vi "execute.vi"(8 "error in (no error)":errorcluster, 10 "ComponentData.lvclass":refnum<class "ComponentData.lvclass">, 11 "OffState in":refnum<class "StandbyState.lvclass">) -> (0 "error out":errorcluster, 2 "ComponentData.lvclass 2":refnum<class "ComponentData.lvclass">, 3 "OffState out":refnum<class "StandbyState.lvclass">)   [LabVIEW 2013, in "ComponentData.lvlib" / "StandbyState.lvclass"]
uses:
  <userlib>/Common/Component/common_application/RT/ComponentData/ComponentState/StandbyState/StandbyState.lvclass
  <userlib>/Common/Component/common_application/RT/ComponentData/ComponentData/ComponentData.lvclass
  <userlib>/Common/Component/common_application/RT/ComponentData/ComponentState/ComponentState/ComponentState.lvclass
  <userlib>/Common/Component/common_application/RT/ComponentData/componentStateValues.ctl
  <userlib>/Common/Component/common_application/RT/ComponentData/ComponentState/DisabledState/DisabledState.lvclass
  <userlib>/Common/Component/common_application/RT/ComponentData/ComponentState/OffState/OffState.lvclass
  <userlib>/Common/Component/common_application/RT/ComponentData/ApplicationHandler/ApplicationHandler.lvclass
  <userlib>/Common/Component/common_application/RT/ComponentData.lvlib
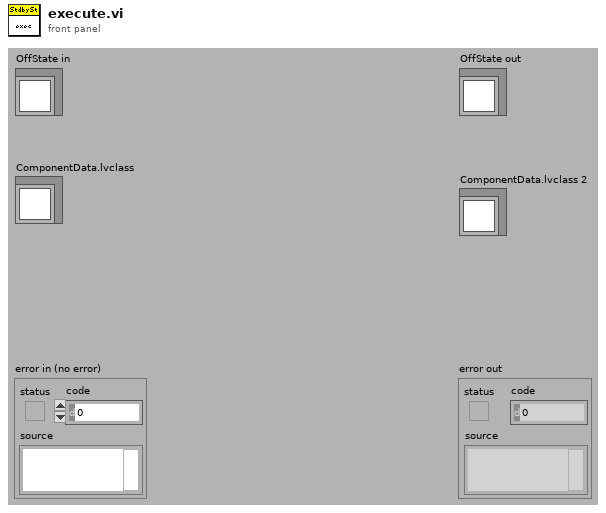
[diagram p1: front panel]
types:
  T1 = typedef "ComponentData.lvlib/componentStateValues.ctl" = enum16{"Off", "Standby", "Enabled", "Disabled", "Fault"}
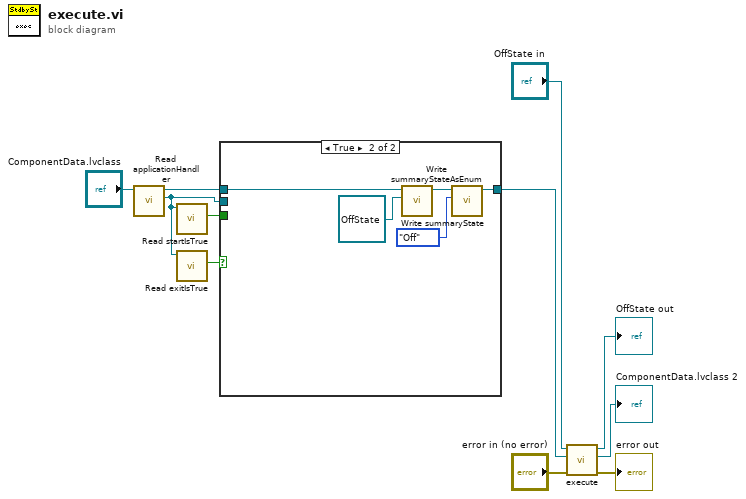
[diagram p0: block diagram]
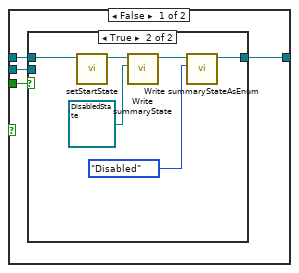
[diagram p2: hidden frame]
diagram:
  n1 = call <userlib>:"Read applicationHandler.vi"("ComponentData in"="ComponentData.lvclass") -> ("ApplicationHandler.lvclass"=w2:refnum<class "ApplicationHandler.lvclass">, "ComponentData out"=w4:refnum<class "ComponentData.lvclass">)  [unwired: 9 in]
  n2 = call <userlib>:"Read startIsTrue.vi"("ApplicationHandler in"=w2) -> ("startIsTrue"=w5:bool)  [unwired: 9 in, 1 out]
  n3 = call <userlib>:"Read exitIsTrue.vi"("ApplicationHandler in"=w2) -> ("exitIsTrue"=w1:bool)  [unwired: 9 in, 1 out]
  n4 = case shown="True" w1 {
    tunnel: w5 -> [w15 _]
    tunnel: w4 -> [w14 w27]
    tunnel: [w13 w25] -> w3
    tunnel: w2 -> [w12 _]
    frame False {
      n5 = case shown="True" w15 {
        tunnel: w14 -> [w16 w18]
        tunnel: [w16 w20] -> w13
        tunnel: w12 -> [_ _]
        frame False {
        }
        frame True {
          n6 = call-dynamic "setStartState.vi"("ComponentData in"=w18) -> ("ComponentData out"=w17:refnum<class "ComponentData.lvclass">)  [unwired: 9 in, 1 out]
          n7 = call <userlib>:"Write summaryState.vi"("ComponentState.lvclass"=refnum<class "DisabledState.lvclass"> refnum ("DisabledState.lvclass"), "ComponentData in"=w17) -> ("ComponentData out"=w22:refnum<class "ComponentData.lvclass">)  [unwired: 9 in]
          n8 = call <userlib>:"Write summaryStateAsEnum.vi"("componentStateValues"=componentStateValues."Disabled", "ComponentData in"=w22) -> ("ComponentData out"=w20:refnum<class "ComponentData.lvclass">)  [unwired: 8 in, 1 out]
        }
      }
    }
    frame True {
      n9 = call <userlib>:"Write summaryState.vi"("ComponentState.lvclass"=refnum<class "OffState.lvclass"> refnum ("UnknownState.lvclass"), "ComponentData in"=w27) -> ("ComponentData out"=w26:refnum<class "ComponentData.lvclass">)  [unwired: 9 in]
      n10 = call <userlib>:"Write summaryStateAsEnum.vi"("componentStateValues"=componentStateValues."Off", "ComponentData in"=w26) -> ("ComponentData out"=w25:refnum<class "ComponentData.lvclass">)  [unwired: 8 in, 1 out]
    }
  }
  n11 = call-parent "execute.vi"("error in (no error)"="error in (no error)", "ComponentData.lvclass"=w3, "ComponentState in"="OffState in") -> ("error out"=→"error out":errorcluster, "ComponentData.lvclass 2"=→"ComponentData.lvclass 2":refnum<class "ComponentData.lvclass">, "ComponentState out"=→"OffState out":refnum<class "StandbyState.lvclass">)  [unwired: 6 in]
